vi "LC Export.vi"(8 "error in (no error)":errorcluster caption="Error In") -> (0 "error out":errorcluster caption="Error Out")   [LabVIEW 2020]
uses:
  LC Mode.ctl
  LC Single Control Information.ctl
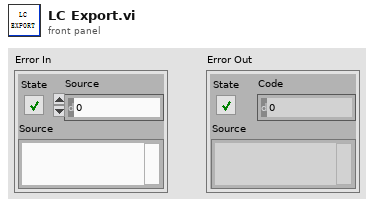
[diagram p1: front panel]
types:
  T1 = typedef "LC Single Control Information.ctl" = cluster{"VI Path":string, "VI Name":string, "Control Name":string, "Property Type":string, "Language":string, "Content":string}
  T2 = typedef "LC Mode.ctl" = enum16{"Init", "NONE", "Read", "Write", "Delete", "Clear", "Save"}
  T3 = typedef "LC Control Information.ctl" = cluster{"Controls":cluster{"Control Name":string, "Property Type":string, "Content":cluster{"Language":string, "Content":string}[]}[], "VI Path":string, "VI Name":string}[]
  T4 = cluster{"Control Name":string, "Property Type":string, "Content":cluster{"Language":string, "Content":string}[]}[]
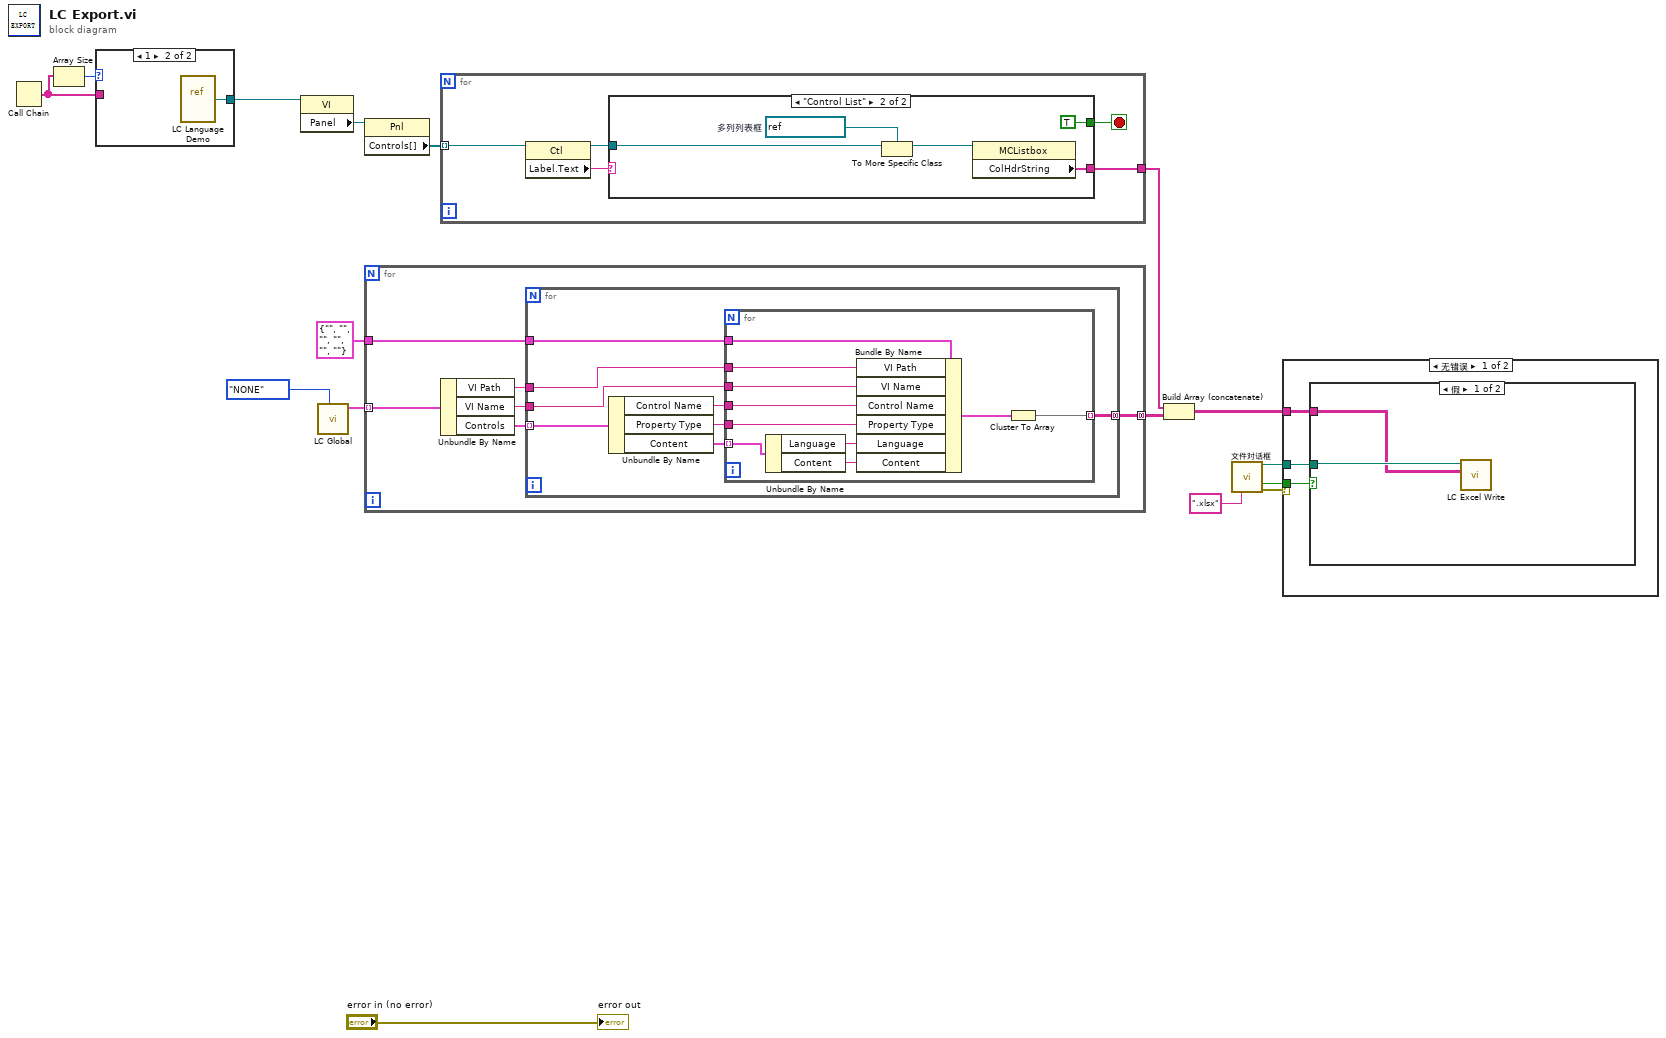
[diagram p0: block diagram]
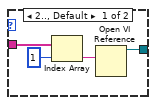
[diagram p5: hidden frame]
diagram:
  n1 = Call Chain() -> (call chain=w13:string[])
  n2 = Array Size(array=w13) -> (size(s)=w14:i32)
  n3 = case shown="1" w14 {
    tunnel: [w18 w21] -> w11
    tunnel: w13 -> [w17 _]
    frame 2.., Default {
      n4 = Index Array(array=w17, index=1 ("索引")) -> (element=w19:string)
      n5 = Open VI Reference(vi path=w19) -> (vi reference=w18:refnum<vi>)  [unwired: 5 in, 1 out]
    }
    frame 1 {
      n6 = vi-ref "LC Language Demo.vi"() -> (w21:refnum<vi>)
    }
  }
  n7 = property class="VI"(reference=w11) -> ("Panel"=w12:refnum<vi>)  [unwired: 1 in, 2 out]
  n8 = call "LC Global.vi"("Mode"=LC_Mode."NONE") -> ("VI Info"=w9:T3)  [unwired: 8 in, 2 out]
  n9 = property class="Pnl"(reference=w12) -> ("Controls[]"=w15:refnum<vi>[])  [unwired: 1 in, 2 out]
  n10 = for {
    tunnel: w9 -> [w27] mode=indexing
    tunnel: T1 {"VI Path"="", "VI Name"="", "Control Name"="", "Property Type"="", "Language"="", "Content"=""} ("Write") -> [w26]
    tunnel: [w22] -> w3 mode=concatenating
    n11 = Unbundle By Name(w27) -> ("VI Path"=w25:string, "VI Name"=w24:string, "Controls"=w23:T4)
    n12 = for {
      tunnel: w26 -> [w35]
      tunnel: w25 -> [w34]
      tunnel: w24 -> [w33]
      tunnel: w23 -> [w32] mode=indexing
      tunnel: [w28] -> w22 mode=concatenating
      n13 = Unbundle By Name(w32) -> ("Control Name"=w31:string, "Property Type"=w30:string, "Content"=w29:cluster{"Language":string, "Content":string}[])
      n14 = for {
        tunnel: w35 -> [w45]
        tunnel: w34 -> [w44]
        tunnel: w33 -> [w43]
        tunnel: w31 -> [w42]
        tunnel: w30 -> [w41]
        tunnel: w29 -> [w40] mode=indexing
        tunnel: [w36] -> w28 mode=indexing
        n15 = Unbundle By Name(w40) -> ("Language"=w39:string, "Content"=w38:string)
        n16 = Bundle By Name(cluster=w45, "VI Path"=w44, "VI Name"=w43, "Control Name"=w42, "Property Type"=w41, "Language"=w39, "Content"=w38) -> (w37:T1)
        n17 = Cluster To Array(cluster=w37) -> (array=w36:string[])
      }
    }
  }
  n18 = for {
    tunnel: w15 -> [w50] mode=indexing
    tunnel: [w46] -> w2
    stop <- w47 stop-if-true
    n19 = property class="Ctl"(reference=w50) -> (reference out=w48:refnum<vi>, "Label.Text"=w49:string)  [unwired: 1 in, 1 out]
    n20 = case shown="\"Control List\"" w49 {
      tunnel: w48 -> [_ w55]
      tunnel: [_ TRUE] -> w47
      tunnel: [_ w51] -> w46
      frame "eee", Default {
      }
      frame "Control List" {
        w53 = refnum<vi> refnum  # 多列列表框
        n21 = To More Specific Class(target class=w53, reference=w55) -> (specific class reference=w54:refnum<vi>)  [unwired: 1 in, 1 out]
        n22 = property class="MCListbox"(reference=w54) -> ("ColHdrString"=w51:string[])  [unwired: 1 in, 2 out]
      }
    }
  }
  n23 = Build Array (concatenate)(w2, w3) -> (w1:string[][])
  n24 = call "文件对话框"("pattern (all files)"=".xlsx") -> ("selected path"=w4:path, "cancelled"=w5:bool, "error out"=w7:errorcluster)  [unwired: 11 in, 1 out]
  n25 = case shown="无错误" w7 {
    tunnel: w5 -> [w58 _]
    tunnel: w4 -> [w57 _]
    tunnel: w1 -> [w56 _]
    frame No Error {
      n26 = case shown="假" w58 {
        tunnel: w57 -> [w60 _]
        tunnel: w56 -> [w59 _]
        frame False {
          n27 = call "LC Excel Write.vi"("Write"=w59, "Path"=w60) -> ()  [unwired: 9 in, 1 out]
        }
        frame True {
        }
      }
    }
    frame Error {
    }
  }
  "error out" <- "error in (no error)"
